vi "Search peak att.vi"(8 "error in":errorcluster, 10 "App Data":T1, 11 "XYGraph in":refnum<vi>) -> (0 "error out":errorcluster)   [LabVIEW 2014]
uses:
  Controls/App Data.ctl
panel:
  in  "index":i32
  out "subarray":dbl[][](array[numeric])
  out "index of min y value":i32
  out "min value = max. atten.":dbl
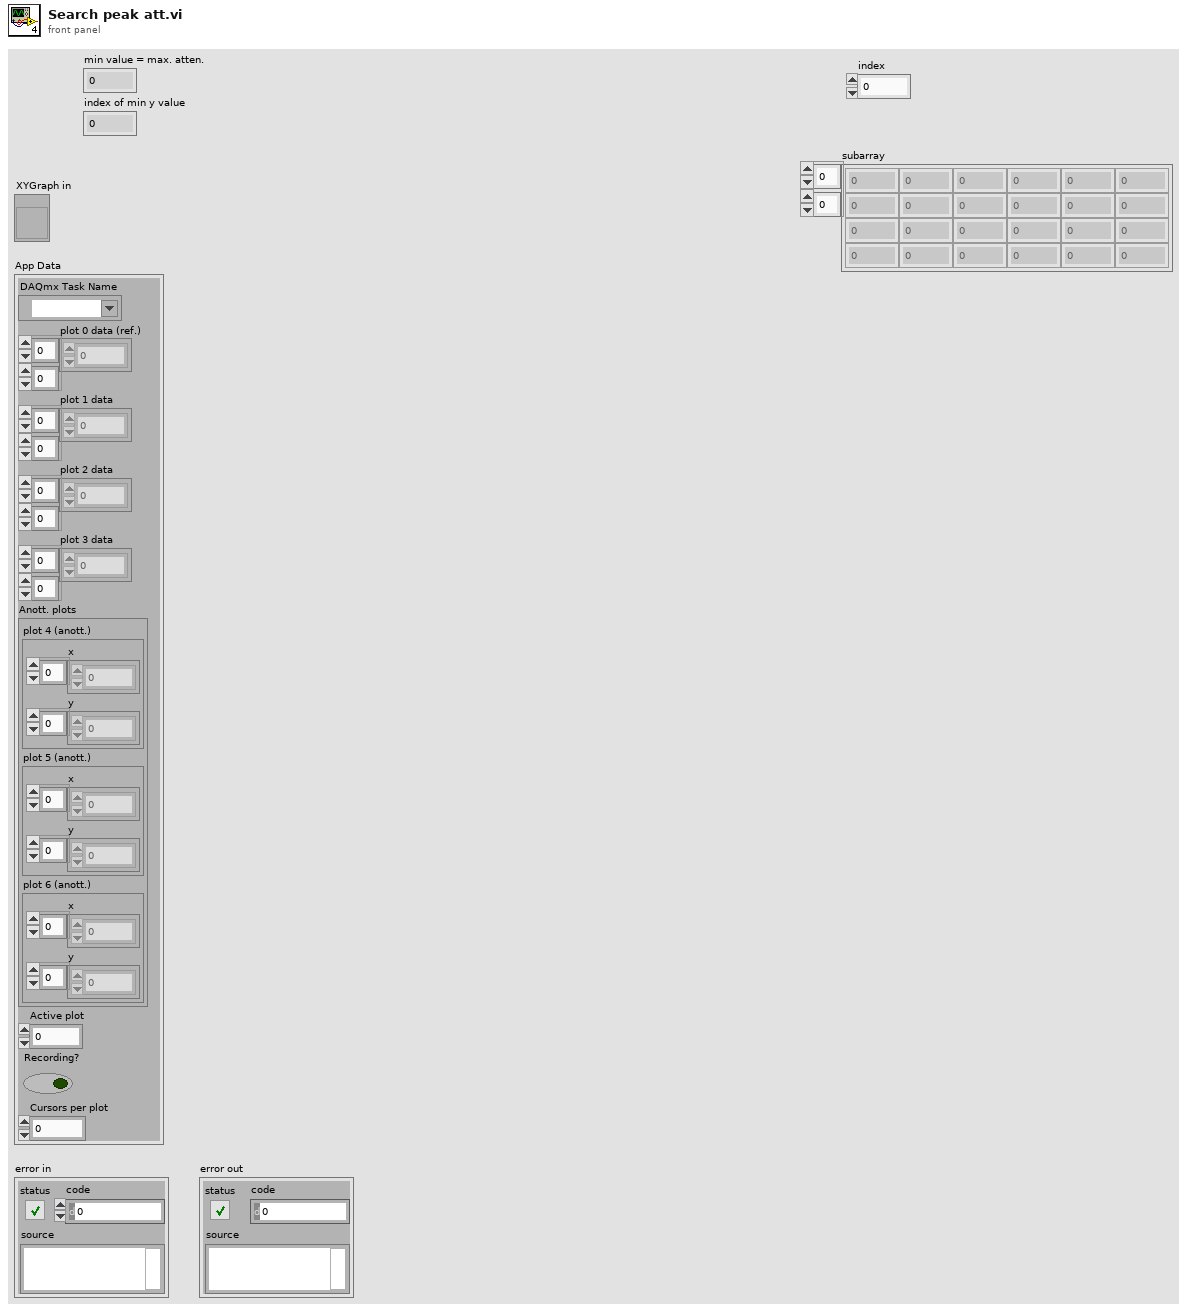
[diagram p1: front panel]
types:
  T1 = typedef "App Data.ctl" = cluster{"DAQmx Task Name":refnum<k21>, "plot 0 data (ref.)":dbl[][], "plot 1 data":dbl[][], "plot 2 data":dbl[][], "plot 3 data":dbl[][], "Anott. plots":cluster{"plot 4 (anott.)":cluster{"x":dbl[], "y":dbl[]}, "plot 5 (anott.)":cluster{"x":dbl[], "y":dbl[]}, "plot 6 (anott.)":cluster{"x":dbl[], "y":dbl[]}}, "Active plot":u32, "Recording?":bool, "Cursors per plot":i32}
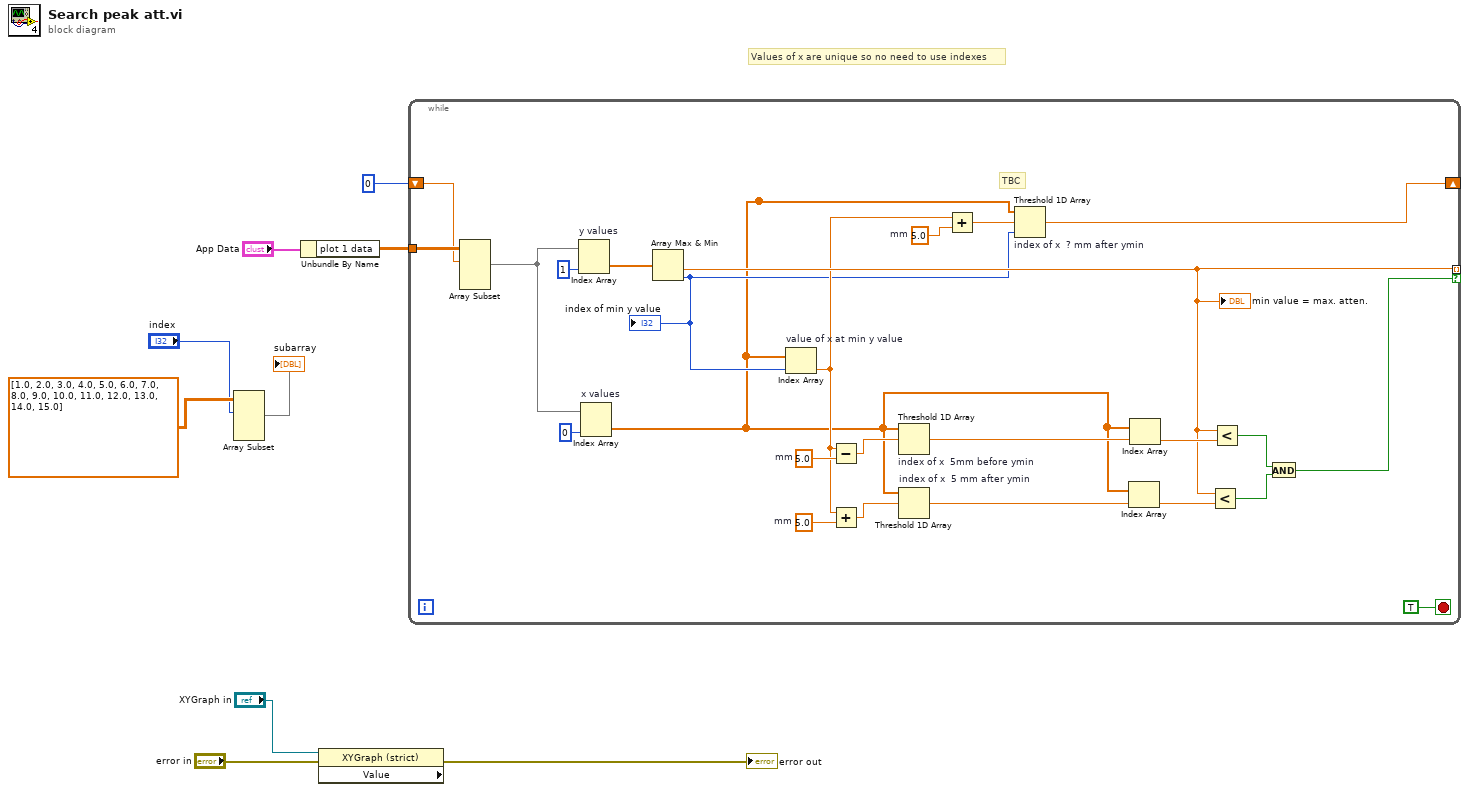
[diagram p0: block diagram]
diagram:
  # "Values of x are unique so no need to use indexes"
  n1 = Array Subset "Array Subset"(array=dbl[][] [[1.0, 2.0, 3.0, 4.0, 5.0], [6.0, 7.0, 8.0, 9.0, 10.0], [11.0, 12.0, 13.0, 14.0, 15.0]], index (row)="index") -> (→"subarray":dbl[][])  [unwired: 3 in]
  n2 = Unbundle By Name("App Data") -> ("plot 1 data"=w5:dbl[][])
  n3 = property class="XYGraph (strict)" props=["Value"](reference="XYGraph in", error in="error in") -> (error out=→"error out":errorcluster)  [unwired: 2 out]
  n4 = while {
    tunnel: w5 -> [w19]
    tunnel: [w21] -> _ mode=indexing if=w20
    shift-right: [w12] -> _
    shift-left: 0 ("index") -> [w16]
    stop <- TRUE stop-if-true
    w15 = 5.0  # mm
    w29 = 5.0  # mm
    w30 = 5.0  # mm
    # "TBC"
    n5 = Array Subset "Array Subset"(array=w19, index (row)=w16) -> (w18:dbl[][])  [unwired: 3 in]
    n6 = Index Array "y values"(array=w18, index (col)=1 ("disabled index (col)")) -> (element=w33:dbl[])  [unwired: 1 in]
    n7 = Index Array "x values"(array=w18, index (col)=0 ("disabled index (col)")) -> (element=w10:dbl[])  [unwired: 1 in]
    n8 = Array Max & Min(array=w33) -> (min value=w21:dbl, min index (indices)=w11:i32)  [unwired: 2 out]
    "min value = max. atten." <- w21
    "index of min y value" <- w11
    n9 = Index Array "value of x at min y value"(array=w10, index=w11) -> (element=w13:dbl)
    n10 = Subtract(x=w13, y=w30) -> (x-y=w31:dbl)
    n11 = Add(x=w13, y=w29) -> (x+y=w28:dbl)
    n12 = Threshold 1D Array "index of x  5mm before ymin"(2:w31, 3:w10) -> (0:w27:dbl)  [unwired: 1 in]
    n13 = Threshold 1D Array "index of x  5 mm after ymin"(2:w28, 3:w10) -> (0:w26:dbl)  [unwired: 1 in]
    n14 = Add(x=w13, y=w15) -> (x+y=w14:dbl)
    n15 = Threshold 1D Array "index of x  ? mm after ymin"(1:w11, 2:w14, 3:w10) -> (0:w12:dbl)
    n16 = Index Array(array=w10, index=w26) -> (element=w24:dbl)
    n17 = Index Array(array=w10, index=w27) -> (element=w25:dbl)
    n18 = Less?(x=w21, y=w24) -> (x < y?=w22:bool)
    n19 = Less?(x=w21, y=w25) -> (x < y?=w23:bool)
    n20 = And(x=w23, y=w22) -> (x .and. y?=w20:bool)
  }
